vi "instrument_IO.vi"() -> ()   [LabVIEW 2017]
panel:
  out "return count":u32
  out "error out":errorcluster
  in  "error in (no error)":errorcluster
  out "read buffer":string
  out "VISA resource name out":refnum<visa-resource-name>
  in  "VISA resource name":refnum<visa-resource-name>
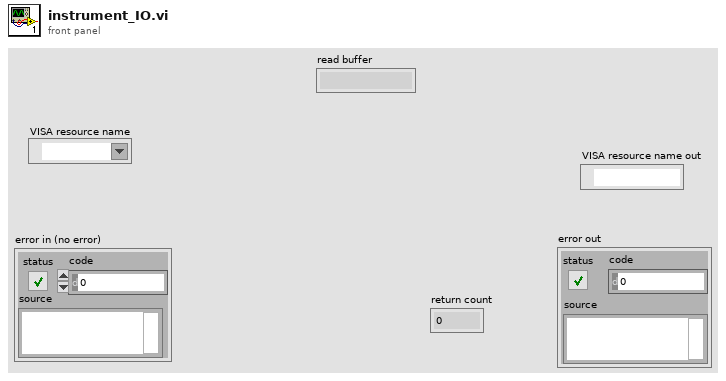
[diagram p1: front panel]
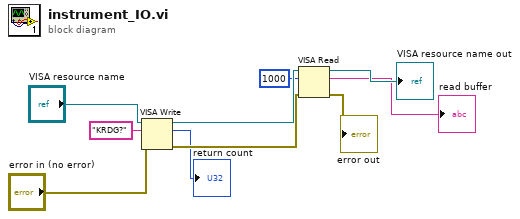
[diagram p0: block diagram]
diagram:
  n1 = VISA Write(VISA resource name="VISA resource name", write buffer="KRDG?", error in (no error)="error in (no error)") -> (VISA resource name out=w9:refnum<visa-resource-name>, return count=→"return count":u32, error out=w4:errorcluster)
  n2 = VISA Read(VISA resource name=w9, byte count=u32 1000, error in (no error)=w4) -> (VISA resource name out=→"VISA resource name out":refnum<visa-resource-name>, read buffer=→"read buffer":string, error out=→"error out":errorcluster)  [unwired: 1 out]
